vi "post_dust_source_small.vi"(8 "error in (no error)":errorcluster, 11 "Dust control settings":T1={"Integer Timestamp"=8, "Needle Voltage"=2.0, "Frequency"=3.0, "Width (ms) : 0.1 "=4.0, "Desired Amplitude (V)"=5.0, "Settings ID"="", "ID#"=7} {"Needle Voltage" min=0.0 max=10.0 step=0.01 format="%.2g"; "Desired Amplitude (V)" min=0.0 max=10.0 step=0.01 format="%5.2f"; "Width (ms) : 0.1" min=0.05 max=5.0 step=0.01 format="%6.2f"; "Frequency" min=1.0 max=100.0 step=0.01 format="%.1f"}) -> (0 "error out":errorcluster)   [LabVIEW 2015]
doc: "Adds a new row to the source_settings table."
uses:
  User Interface/Controls/dust_source_control_small.ctl
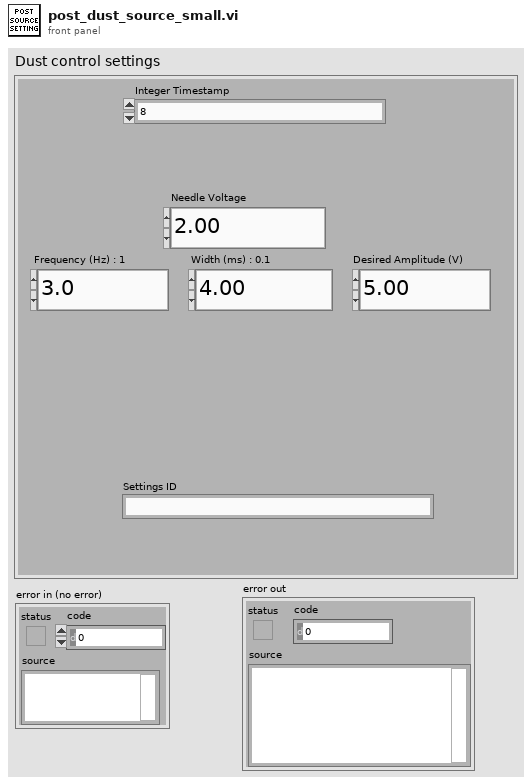
[diagram p1: front panel]
types:
  T1 = typedef "dust_source_control_small.ctl" = cluster{"Integer Timestamp":u64, "Needle Voltage":dbl, "Frequency":dbl, "Width (ms) : 0.1 ":dbl, "Desired Amplitude (V)":dbl, "Settings ID":string, "ID#":i32}
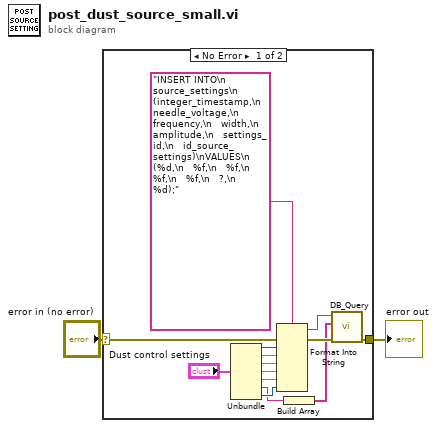
[diagram p0: block diagram]
diagram:
  n1 = case shown="No Error" "error in (no error)" {
    selector: "error in (no error)" -> [w16 w17]
    tunnel: [w10 w17] -> w1
    frame No Error {
      n2 = Unbundle("Dust control settings") -> ("Integer Timestamp"=w13:u64, "Needle Voltage"=w9:dbl, "Frequency"=w8:dbl, "Width (ms) : 0.1"=w7:dbl, "Desired Amplitude (V)"=w6:dbl, "Settings ID"=w4:string, "ID#"=w5:i32)
      n3 = Format Into String(format string="INSERT INTO\n  source_settings\n  (integer_timestamp,\n   needle_voltage,\n   frequency,\n   width,\n   amplitude,\n   settings_id,\n   id_source_settings)\nVALUES\n  (%d,\n   %f,\n   %f,\n   %f,\n   %f,\n   ?,\n   %d);" ("table"), error in=w16, w13, w9, w8, w7, w6, w5) -> (resulting string=w12:string, error out=w15:errorcluster)  [unwired: 1 in]
      n4 = Build Array(w4) -> (w3:string[])
      n5 = call "DB_Query.vi"("error in (no error)"=w15, "Parameters"=w3, "Parameterized Query"=w12) -> ("error out"=w10:errorcluster)  [unwired: 6 in, 2 out]
    }
    frame Error {
    }
  }
  "error out" <- w1
